vi "Get Measurements.vi"(0 "input path":path, 5 "lab view version":string, 11 "error in":errorcluster) -> (3 "error?":string, 4 "vi list":T1[](array[typedef]), 6 "folder list":T1[](array[typedef]), 15 "error out":errorcluster)   [LabVIEW 2021, in "Converter.lvlib"]
uses:
  Converter.lvlib
  TypeDefs/Multiple Conversion/Tree Items.ctl
  Path Functions/Path Functions.lvlib
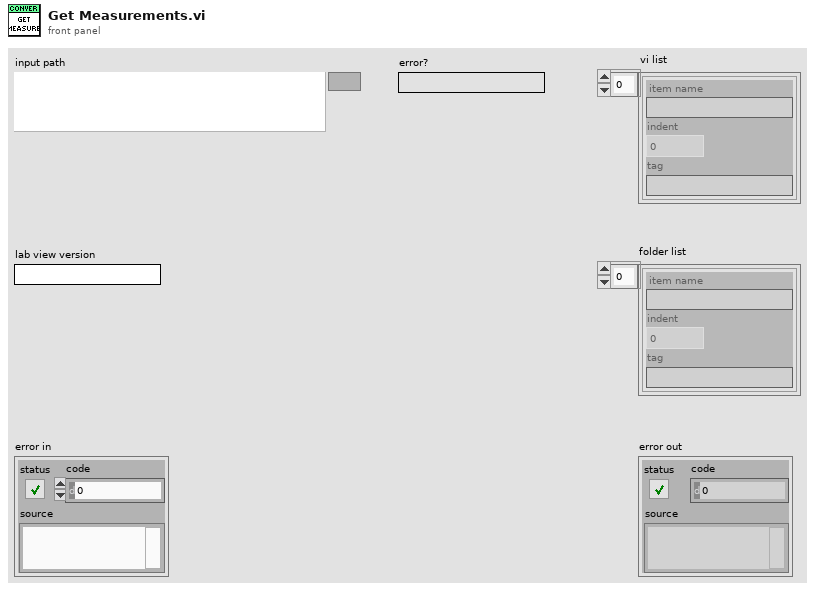
[diagram p1: front panel]
types:
  T1 = typedef "Converter.lvlib/Tree Items.ctl" = cluster{"item name":string, "indent":i32, "tag":string}
  T2 = enum16{"open", "replace", "create", "open or create", "replace or create", "replace or create with confirmation"}
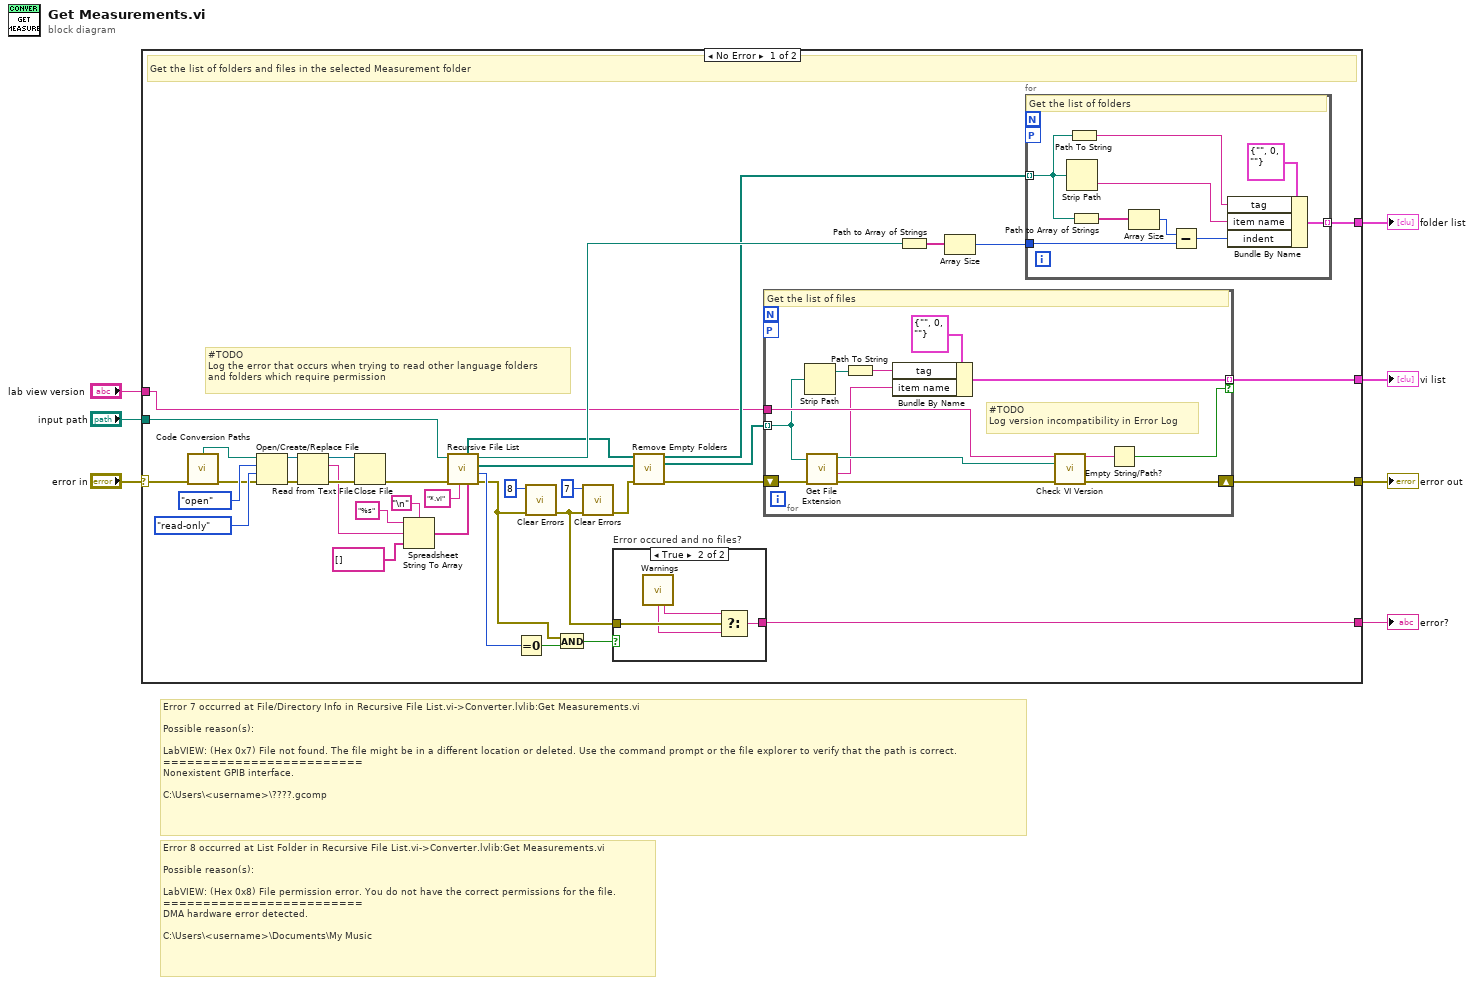
[diagram p0: block diagram]
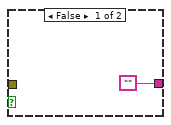
[diagram p2: hidden frame]
diagram:
  # "Error 8 occurred at List Folder in Recursive File List.vi->Converter.lvlib:Get Measurements.vi\n\nPossible reason(s):\n\nLabVIEW: (Hex 0x8) File permission error. You do not have the correct permissions for the file.\n=========================\nDMA hardware error detected.\n\nC:\\Users\\<username>\\Documents\\My Music"
  # "Error 7 occurred at File/Directory Info in Recursive File List.vi->Converter.lvlib:Get Measurements.vi\n\nPossible reason(s):\n\nLabVIEW: (Hex 0x7) File not found. The file might be in a different location or deleted. Use the command prompt or the file explorer to verify that the path is correct.\n=========================\nNonexistent GPIB interface.\n\nC:\\Users\\<username>\\????.gcomp"
  n1 = case shown="No Error" "error in" {
    selector: "error in" -> [w16 w73]
    tunnel: "input path" -> [w40 _]
    tunnel: [w42 w73] -> w5
    tunnel: [w43 _] -> w4
    tunnel: [w41 _] -> w3
    tunnel: "lab view version" -> [w22 _]
    tunnel: [w8 _] -> w1
    frame No Error {
      # "#TODO\nLog the error that occurs when trying to read other language folders \nand folders which require permission"
      # "Get the list of folders and files in the selected Measurement folder"
      n2 = call "Code Conversion Paths.vi"("error in"=w16) -> ("folders to ignore"=w17:path, "error out"=w15:errorcluster)  [unwired: 6 in, 7 out]
      n3 = Open/Create/Replace File(file path (use dialog)=w17, error in=w15, operation (0:open)=T2."open", access (0:read/write)=enum16{"read/write", "read-only", "write-only"}."read-only") -> (refnum out=w30:refnum<file>, error out=w29:errorcluster)  [unwired: 2 in, 1 out]
      n4 = Read from Text File(file (use dialog)=w30, error in=w29) -> (refnum out=w32:refnum<file>, text=w20:string, error out=w31:errorcluster)  [unwired: 2 in, 1 out]
      n5 = Close File(refnum=w32, error in=w31) -> (error out=w23:errorcluster)  [unwired: 1 out]
      n6 = Spreadsheet String To Array(delimiter (Tab)="\n", format string="%s", spreadsheet string=w20, array type (2D Dbl)=string[] []) -> (array=w21:string[])
      n7 = call <vilib>:"Recursive File List.vi"("Folders to Exclude"=w21, "pattern"="*.vi", "error in (no error)"=w23, "Folder Path"=w40) -> ("error out"=w11:errorcluster, "Number of Files"=w13:i32, "All Files in Dir"=w35:path[], "dup Folder Path"=w44:path, "All Folders"=w34:path[])  [unwired: 3 in]
      n8 = Equal To 0?(x=w13) -> (x = 0?=w12:bool)
      n9 = call <vilib>:"Clear Errors.vi"("error in (no error)"=w11, "specific error code to clear (0: all)"=8) -> ("error out"=w9:errorcluster)  [unwired: 4 in, 1 out]
      n10 = And(x=w11, y=w12) -> (x .and. y?=w10:bool)
      n11 = call <vilib>:"Clear Errors.vi"("error in (no error)"=w9, "specific error code to clear (0: all)"=7) -> ("error out"=w14:errorcluster)  [unwired: 4 in, 1 out]
      n12 = case "Error occured and no files?" shown="True" w10 {
        tunnel: w9 -> [_ w50]
        tunnel: ["" w47] -> w8
        frame False {
        }
        frame True {
          n13 = call "Warnings.vi"() -> ("permission error"=w48:string, "invalid folder/file names"=w49:string)  [unwired: 8 in, 6 out]
          n14 = Select(t=w49, s=w50, f=w48) -> (s? t:f=w47:string)
        }
      }
      n15 = call "Remove Empty Folders.vi"("folders path"=w34, "files path"=w35, "error in"=w14) -> ("required folders list"=w36:path[], "files path out"=w33:path[], "error out"=w37:errorcluster)  [unwired: 10 in]
      n16 = for {
        tunnel: [w60] -> w43 mode=indexing if=w54
        shift-right: [w57] -> w42
        shift-left: w37 -> [w59]
        tunnel: w22 -> [w56]
        workers-P: _ -> [_]
        tunnel: w33 -> [w51] mode=indexing
        # "#TODO\nLog version incompatibility in Error Log"
        # "Get the list of files"
        n17 = Strip Path(path=w51) -> (stripped path=w63:path)  [unwired: 1 out]
        n18 = call <vilib>:"Get File Extension.vi"("error in (no error)"=w59, "file"=w51) -> ("error out"=w58:errorcluster, "filename without extension"=w53:string, "dup file"=w55:path)  [unwired: 5 in, 2 out]
        n19 = Path To String(path=w63) -> (string=w61:string)
        n20 = Bundle By Name(cluster=T1 {"item name"="", "indent"=0, "tag"=""} ("Cluster"), "tag"=w61, "item name"=w53) -> (w60:T1)
        n21 = call "Check VI Version.vi"("lab view version"=w56, "vi path"=w55, "error in"=w58) -> ("incompatible version warning"=w52:string, "error out"=w57:errorcluster)  [unwired: 11 in]
        n22 = Empty String/Path?(string/path=w52) -> (empty?=w54:bool)
      }
      n23 = Path to Array of Strings(0:w44) -> (2:w45:string[])  [unwired: 1 out]
      n24 = Array Size(array=w45) -> (size(s)=w39:i32)
      n25 = for {
        tunnel: w39 -> [w70]
        tunnel: [w67] -> w41 mode=indexing
        workers-P: _ -> [_]
        tunnel: w36 -> [w64] mode=indexing
        # "Get the list of folders"
        n26 = Strip Path(path=w64) -> (name=w68:string)  [unwired: 1 out]
        n27 = Path To String(path=w64) -> (string=w66:string)
        n28 = Path to Array of Strings(0:w64) -> (2:w72:string[])  [unwired: 1 out]
        n29 = Array Size(array=w72) -> (size(s)=w71:i32)
        n30 = Subtract(x=w71, y=w70) -> (x-y=w65:i32)
        n31 = Bundle By Name(cluster=T1 {"item name"="", "indent"=0, "tag"=""} ("Cluster"), "tag"=w66, "item name"=w68, "indent"=w65) -> (w67:T1)
      }
    }
    frame Error {
      # "Pass"
    }
  }
  "error out" <- w5
  "folder list" <- w3
  "vi list" <- w4
  "error?" <- w1
